vi "_PC_Pub_Dialog_XYGraph.vi"(7 "signal in":waveform(sgl), 8 "error in (no error)":errorcluster) -> (0 "error out":errorcluster)   [LabVIEW 2018]
uses:
  Class/Sig2MS/Sig2MS.lvclass
panel:
  in  "XY Graph":cluster{dbl[], sgl[]}[](graph)
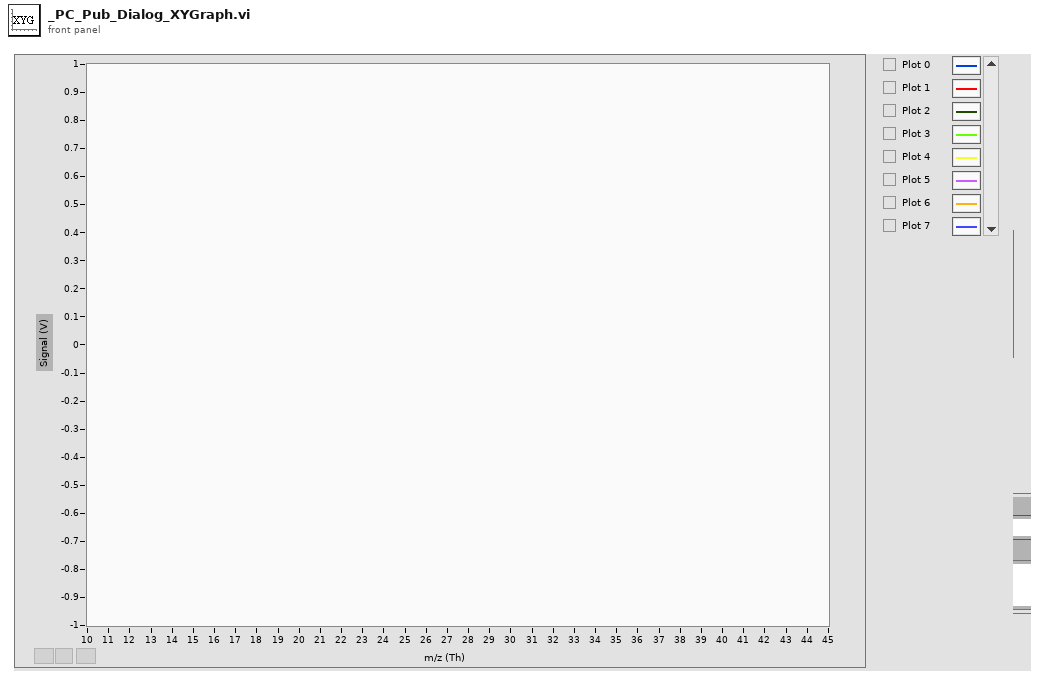
[diagram p1: front panel]
types:
  T1 = enum16{"init", "loadScript", "newScript", "runScript", "close"}
  T2 = enum32{"Invalid", "Default", "Floating", "Floating/Auto-Hide", "Modal"}
  T3 = cluster{"startTime":dbl, "scanSig":cluster{"priDt":dbl, "priXData":dbl[], "priYData":sgl[], "beta":dbl[]}[], "ionSig":cluster{"secDt":dbl, "secYData":sgl[]}[]}
  T4 = cluster{"startTime":dbl, "scanData":cluster{"dt":dbl, "xdata":dbl[], "ydata":sgl[], "beta":dbl[]}[], "xyXLabel":string, "xyYLabel":string, "wfmXLabel":string, "wfmYLabel":string, "ionData":cluster{"dt":dbl, "ydata":sgl[]}[], "ionXLabel":string, "ionYLabel":string}
  T5 = cluster{"dt":dbl, "xdata":dbl[], "ydata":sgl[], "beta":dbl[]}[]
  T6 = cluster{"BGColor":u32, "GridX":bool, "GridY":bool, "LineColorArray":u32[], "LineWidthArray":u8[]}
  T7 = typedef "eventvkey.ctl" = enum16{"ASCII", "Enter", "Return", "Shift", "Ctrl", "Alt", "Cmd", "Opt", "Caps", "NumLock", "Clear", "Break", "Up", "Down", "Left", "Right", "Insert", "Delete", "Home", "End", "PageUp", "PageDown", "Escape", "Help", "Pause", "ScrollLock", "F1", "F2", "F3", "F4", "F5", "F6", "F7", "F8", "F9", "F10", "F11", "F12", "F13", "F14", "F15", "F16", "F17", "F18", "F19", "F20", "F21", "F22", "F23", "F24", "Play", "VolumeUp", "VolumeDown", "Mute", "Two Byte Char"}
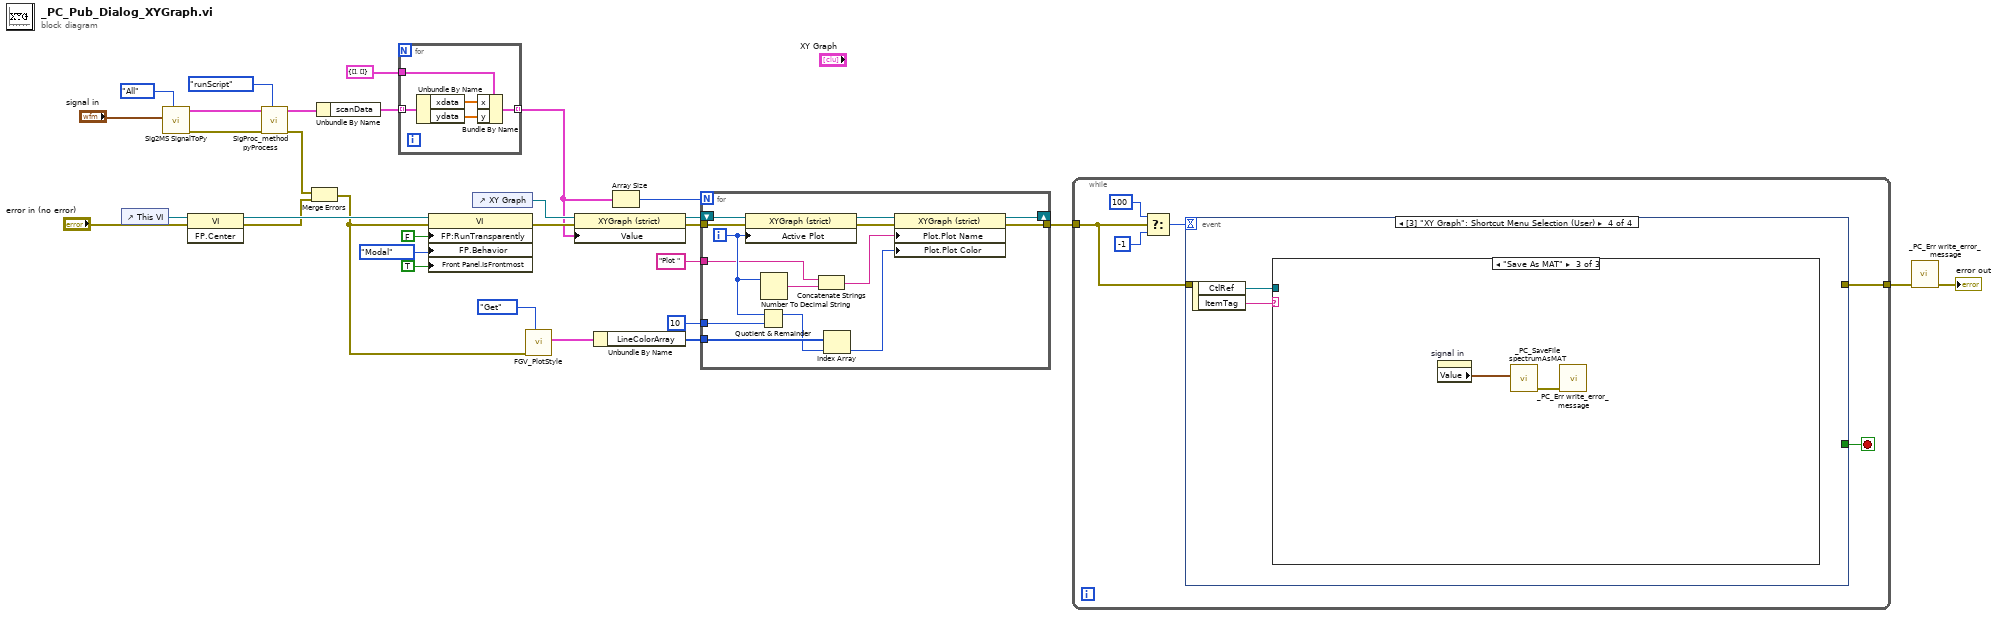
[diagram p0: block diagram]
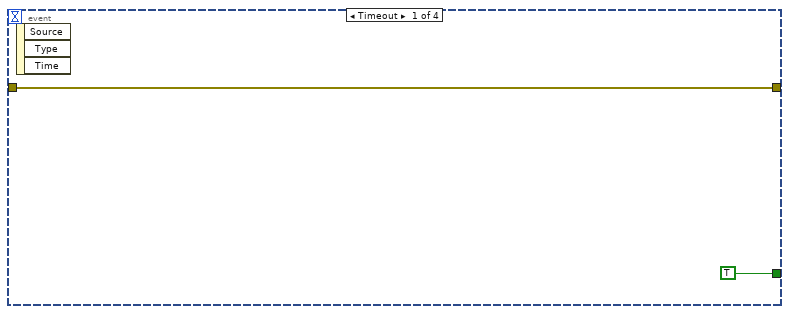
[diagram p2: hidden frame]
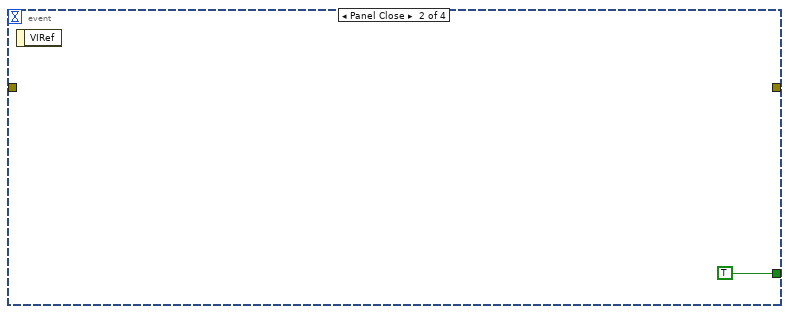
[diagram p3: hidden frame]
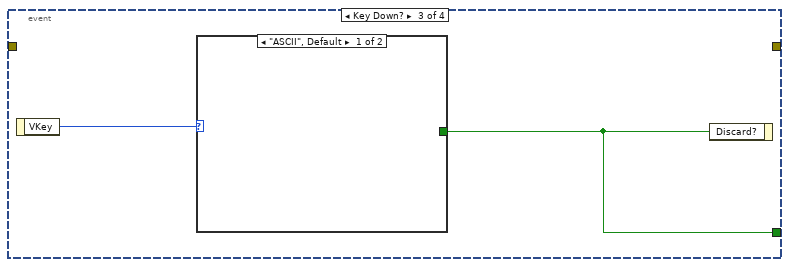
[diagram p4: hidden frame]
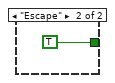
[diagram p5: hidden frame]
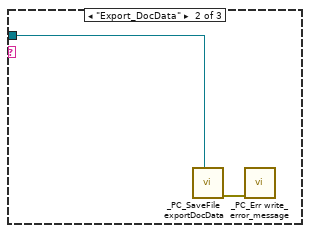
[diagram p7: hidden frame]
diagram:
  n1 = control-ref of="This VI"() -> (w27:refnum<vi>)
  n2 = call "Sig2MS SignalToPy.vi"("getType"=enum16{"All", "Spectra", "Ionisation"}."All", "rawSignal"="signal in") -> ("error out"=w12:errorcluster, "pySigFormat"=w13:T3)  [unwired: 8 in]
  n3 = invoke class="VI" method="FP.Center"(reference=w27, error in="error in (no error)") -> (reference out=w28:refnum<vi>, error out=w4:errorcluster)  [unwired: 1 in, 1 out]
  n4 = call "SigProc_method pyProcess.vi"("func"=T1."runScript", "error in (no error)"=w12, "dataParam"=w13) -> ("error out"=w5:errorcluster, "newSigInfo"=w9:T4)  [unwired: 5 in, 2 out]
  n5 = Merge Errors(w5, w4) -> (w3:errorcluster)
  n6 = Unbundle By Name(w9) -> ("scanData"=w8:T5)
  n7 = for {
    tunnel: w8 -> [w36] mode=indexing
    tunnel: cluster{"x":dbl[], "y":sgl[]} {"x"=[], "y"=[]} -> [w35]
    tunnel: [w32] -> w6 mode=indexing
    n8 = Unbundle By Name(w36) -> ("xdata"=w34:dbl[], "ydata"=w33:sgl[])
    n9 = Bundle By Name(cluster=w35, "x"=w34, "y"=w33) -> (w32:cluster{"x":dbl[], "y":sgl[]})
  }
  n10 = property class="VI"(reference=w28, error in=w3, "FP:RunTransparently"=FALSE ("Front Panel Window:Run VI Transparently"), "FP.Behavior"=T2."Modal" ("Front Panel Window:Behavior"), "Front Panel.IsFrontmost"=TRUE ("Front Panel Window:Is Frontmost")) -> (error out=w16:errorcluster)  [unwired: 1 out]
  n11 = control-ref of="XY Graph"() -> (w17:refnum<vi>)
  n12 = call "FGV_PlotStyle.vi"("Function"=enum16{"Set", "Get"}."Get", "error in (no error)"=w3) -> ("Output Cluster"=w24:T6)  [unwired: 8 in, 1 out]
  n13 = property class="XYGraph (strict)"(reference=w17, error in=w16, "Value"=w6) -> (reference out=w15:refnum<vi>, error out=w14:errorcluster)
  n14 = Unbundle By Name(w24) -> ("LineColorArray"=w23:u32[])
  n15 = Array Size(array=w6) -> (size(s)=w20:i32)
  n16 = for {
    N: w20 -> [_]
    tunnel: [w47] -> w2
    tunnel: w23 -> [w44]
    tunnel: 10 -> [w45]
    tunnel: w14 -> [w41]
    tunnel: "Plot " ("Plot.Plot Name") -> [w38]
    shift-right: [w48] -> _
    shift-left: w15 -> [w50]
    i -> [w40]
    n17 = property class="XYGraph (strict)"(reference=w50, error in=w41, "Active Plot"=w40) -> (reference out=w49:refnum<vi>, error out=w46:errorcluster)
    n18 = Quotient & Remainder(x=w40, y=w45) -> (x-y*floor(x/y)=w42:i32)  [unwired: 1 out]
    n19 = Number To Decimal String(number=w40) -> (decimal integer string=w39:string)  [unwired: 1 in]
    n20 = Concatenate Strings(w38, w39) -> (w37:string)
    n21 = Index Array(array=w44, index=w42) -> (element=w43:u32)
    n22 = property class="XYGraph (strict)"(reference=w49, error in=w46, "Plot.Plot Name"=w37, "Plot.Plot Color"=w43) -> (reference out=w48:refnum<vi>, error out=w47:errorcluster)
  }
  n23 = while {
    tunnel: w2 -> [w52]
    tunnel: [w51] -> w19
    stop <- w56 stop-if-true
    n24 = Select(t=100, s=w52, f=-1) -> (s? t:f=w53:i32)
    n25 = event shown="[3] \"XY Graph\": Shortcut Menu Selection (User)" {
      selector: _ -> [_ _ _ _]
      dyn-events: _ -> [_ _ _ _]
      timeout: w53 -> [_ _ _ _]
      tunnel: [TRUE TRUE w60 _] -> w56
      tunnel: w52 -> [w57 _ _ _]
      tunnel: [w57 _ _ _] -> w51
      event Timeout {
        n26 = event-data() -> ()  [unwired: 1 in, 3 out]
      }
      event Panel Close {
        n27 = event-data() -> ()  [unwired: 1 in, 1 out]
      }
      event Key Down? {
        n28 = event-data() -> ("VKey"=w61:T7)  [unwired: 1 in]
        n29 = case shown="\"ASCII\", Default" w61 {
          tunnel: [_ TRUE] -> w60
          frame "ASCII", Default {
          }
          frame "Escape" {
          }
        }
        n30 = event-data("Discard?"=w60) -> ()  [unwired: 1 in, 1 out]
      }
      event "XY Graph": Shortcut Menu Selection (User) {
        n31 = event-data() -> ("CtlRef"=w64:refnum<vi>, "ItemTag"=w63:string)  [unwired: 1 in]
        n32 = case shown="\"Save As MAT\"" w63 {
          tunnel: w64 -> [_ w66 _]
          frame Default {
          }
          frame "Export_DocData" {
            n33 = call "_PC_SaveFile exportDocData.vi"("xy graph ref"=w66) -> ("error out"=w65:errorcluster)  [unwired: 10 in]
            n34 = call "_PC_Err write_error_message.vi"("error in"=w65) -> ()  [unwired: 10 in, 1 out]
          }
          frame "Save As MAT" {
            n35 = property on="signal in" class="WFD (strict)"() -> ("Value"=w67:waveform(sgl))  [unwired: 2 in, 2 out]
            n36 = call "_PC_SaveFile spectrumAsMAT.vi"("Spectrum data in"=w67) -> ("error out"=w68:errorcluster)  [unwired: 10 in]
            n37 = call "_PC_Err write_error_message.vi"("error in"=w68) -> ()  [unwired: 10 in, 1 out]
          }
        }
      }
    }
  }
  n38 = call "_PC_Err write_error_message.vi"("error in"=w19) -> ("error out"=→"error out":errorcluster)  [unwired: 10 in]
